vi "Request Data.vi"(10 "Data Request":T3, 11 "Historian Module in":refnum<class "Historian Module.lvclass">) -> (2 "History Data":T1, 3 "Historian Module out":refnum<class "Historian Module.lvclass">)   [LabVIEW 2020, in "VolatusHistorian.lvlib" / "Historian Module.lvclass"]
uses:
  Historian Module.lvclass
  Historian Module.lvclass/Historian Module.ctl
  Data Request.ctl
  VolatusHistorian.lvlib
  Channel History.ctl
  History Data.ctl
panel:
  out "Unknown Channels":string[](array[string])
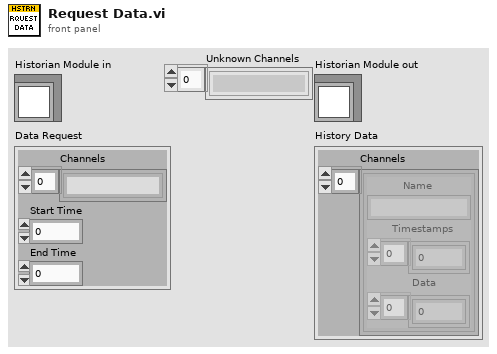
[diagram p1: front panel]
types:
  T1 = typedef "VolatusHistorian.lvlib/History Data.ctl" = cluster{"Channels":T2[]}
  T2 = typedef "VolatusHistorian.lvlib/Channel History.ctl" = cluster{"Name":string, "Timestamps":i64[], "Data":dbl[]}
  T3 = typedef "VolatusHistorian.lvlib/Data Request.ctl" = cluster{"Channels":string[], "Start Time":dbl, "End Time":dbl}
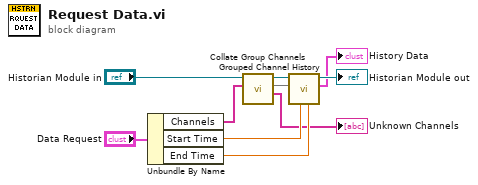
[diagram p0: block diagram]
diagram:
  n1 = Unbundle By Name("Data Request") -> ("Channels"=w8:string[], "Start Time"=w4:dbl, "End Time"=w3:dbl)
  n2 = call "Collate Group Channels.vi"("Channel Names"=w8, "Historian Module in"="Historian Module in") -> ("Unknown Channels"=→"Unknown Channels":string[], "Grouped Channels"=w5:map{string, string[]}, "Historian Module out"=w7:refnum<class "Historian Module.lvclass">)  [unwired: 7 in]
  n3 = call "Grouped Channel History.vi"("End"=w3, "Start"=w4, "Grouped Channels"=w5, "Historian Module in"=w7) -> ("History Data"=→"History Data":T1, "Historian Module out"=→"Historian Module out":refnum<class "Historian Module.lvclass">)  [unwired: 6 in]
